vi "Periodic Tasks.vi"(8 "error in":errorcluster) -> ()   [LabVIEW 2013]
doc: "This VI runs in parallel to other tasks. It can contain as many user-defined periodic loops as you need. These can carry out PID or other sorts of timed response."
uses:
  <vilib>/Rock Robotics/SystemInterfaces/Utilities/FPGA_UtilitiesLED Source.ctl
  <vilib>/Rock Robotics/SystemInterfaces/Utilities/FPGA_UtilitiesLED State.ctl
  Robot Global Data.vi
panel:
  out "Value 2":bool
  out "Value":bool
  out "RDistance":dbl
  out "LDistance":dbl
  out "Distance":dbl
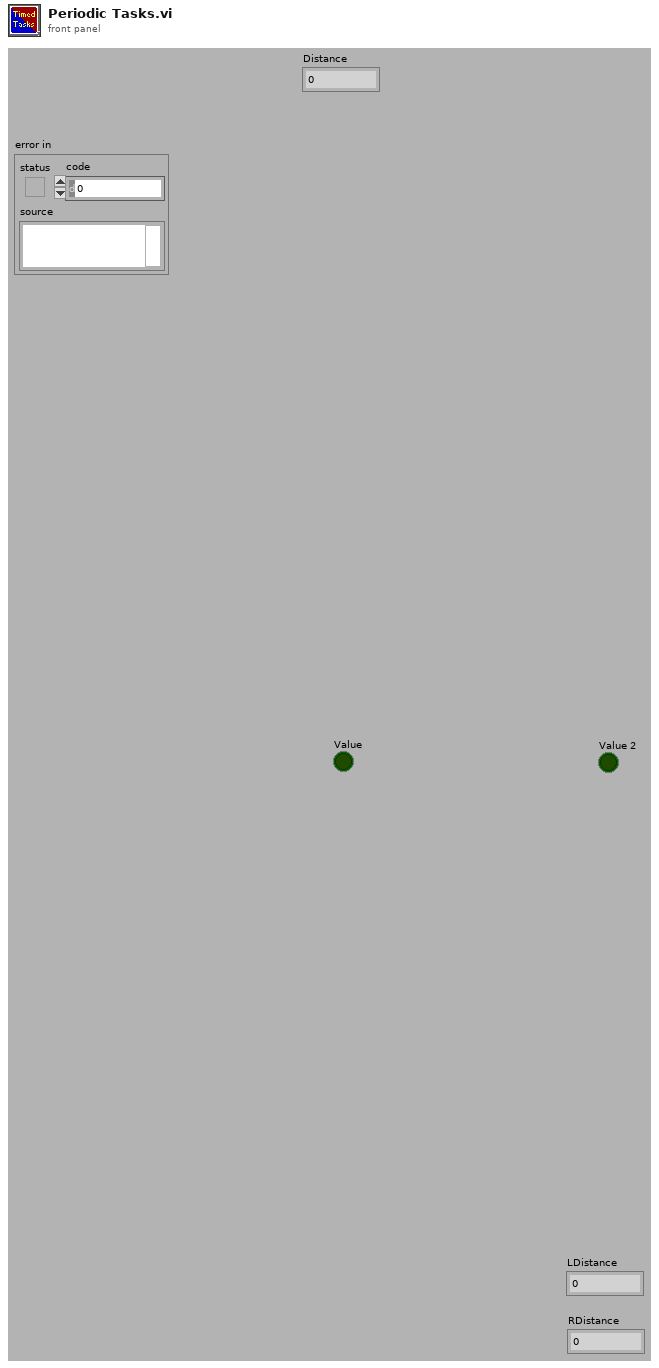
[diagram p1: front panel]
types:
  T1 = typedef "WPI_DigitalInputDevRef.ctl" = cluster{"DevStatus":errorcluster, "DIO Channel":T2, "Digital Module":T3}
  T2 = typedef "FPGA_DIOChannel.ctl" = enum8{"DIO 1", "DIO 2", "DIO 3", "DIO 4", "DIO 5", "DIO 6", "DIO 7", "DIO 8", "DIO 9", "DIO 10", "DIO 11", "DIO 12", "DIO 13", "DIO 14", "Invalid"}
  T3 = typedef "FPGA_TypedefDigitalModule.ctl" = enum16{"Digital Module 1", "Digital Module 2"}
  T4 = typedef "WPI_AnalogChannelDevRef.ctl" = cluster{"DevStatus":errorcluster, "Analog Module":T5, "Analog Channel":T6}
  T5 = typedef "FPGA_TypedefAnalogModule.ctl" = enum16{"Analog Module 1", "Analog Module 2"}
  T6 = typedef "FPGA_AIChannel.ctl" = enum8{"AI 1", "AI 2", "AI 3", "AI 4", "AI 5", "AI 6", "AI 7", "AI 8", "Invalid"}
  T7 = typedef "WPI_EncoderDevRef.ctl" = cluster{"DevStatus":errorcluster, "EncoderIndex":T8, "CounterIndex":T9, "DistancePerCount":dbl, "Decoding Type":T10}
  T8 = typedef "FPGA_EncoderIdx.ctl" = enum8{"Enc 0", "Enc 1", "Enc 2", "Enc 3", "Invalid"}
  T9 = typedef "FPGA_CounterCtrSystemIndex.ctl" = enum8{"Ctr 0", "Ctr 1", "Ctr 2", "Ctr 3", "Ctr 4", "Ctr 5", "Ctr 6", "Ctr 7", "Invalid"}
  T10 = typedef "WPI_EncoderType.ctl" = enum16{"1x", "2x", "4x"}
  T11 = cluster{"Winch Desired Location":dbl, "Winch Desired Location 2":dbl, "Winch Desired Location 3":dbl}
  T12 = typedef "FPGA_UtilitiesLED State.ctl" = enum16{"Off", "On", "Toggle"}
  T13 = typedef "FPGA_UtilitiesLED Source.ctl" = enum16{"User LED", "FPGA LED"}
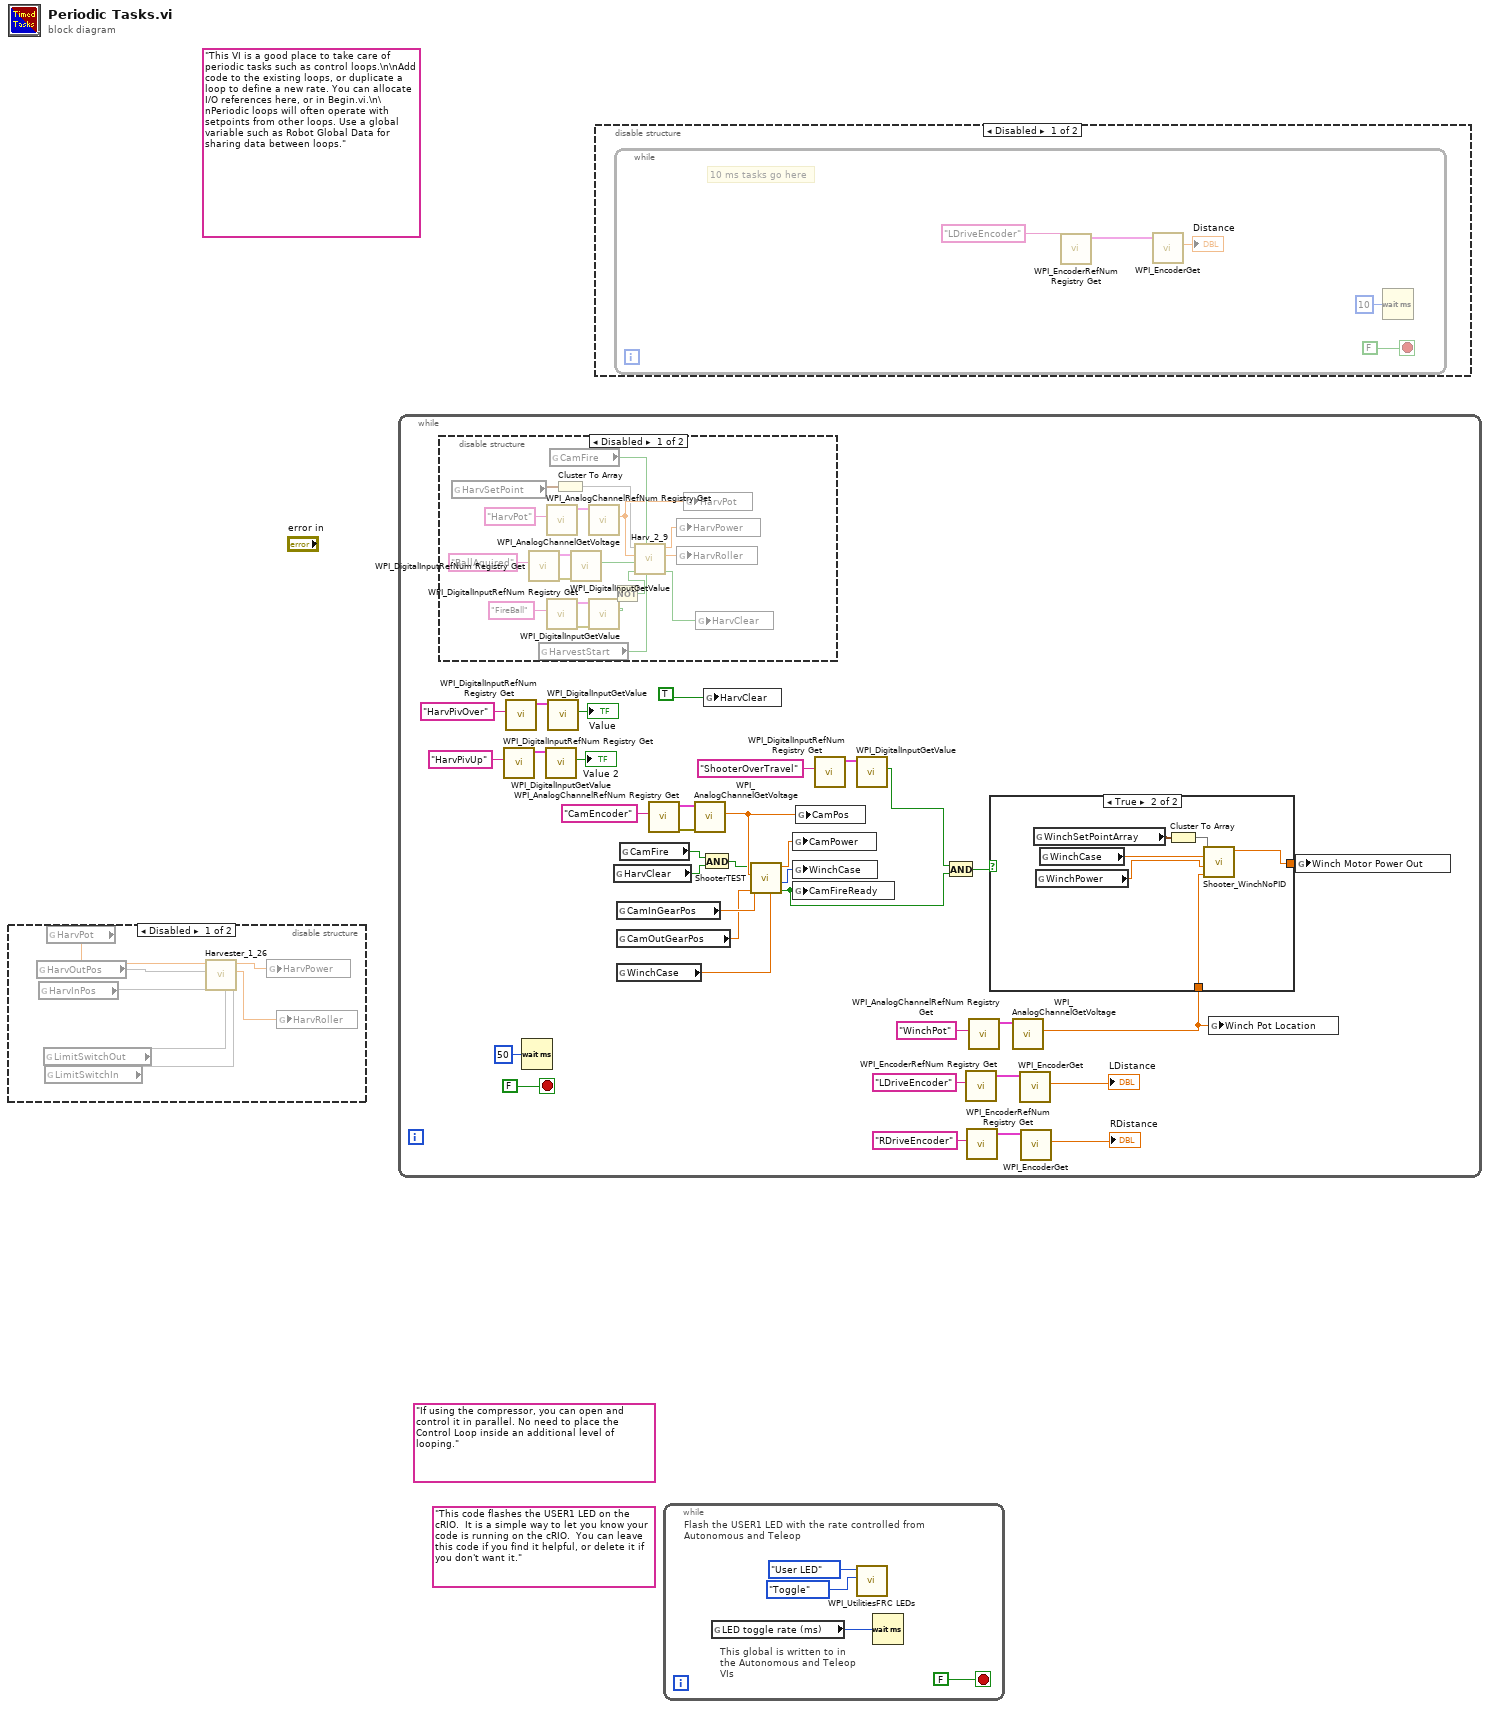
[diagram p0: block diagram]
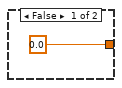
[diagram p5: hidden frame]
diagram:
  (unwired) "If using the compressor, you can open and control it in parallel. No need to place the Control Loop inside an additional level of looping."
  (unwired) "This code flashes the USER1 LED on the cRIO.  It is a simple way to let you know your code is running on the cRIO.  You can leave this code if you find it helpful, or delete it if you don't want it."
  (unwired) "This VI is a good place to take care of periodic tasks such as control loops.\n\nAdd code to the existing loops, or duplicate a loop to define a new rate. You can allocate I/O references here, or in Begin.vi.\n\nPeriodic loops will often operate with setpoints from other loops. Use a global variable such as Robot Global Data for sharing data between loops."
  n1 = disable-structure shown="Disabled" {
    frame Disabled {
      n2 = global read "Robot Global Data.vi" "HarvOutPos"() -> (w6)
      n3 = global read "Robot Global Data.vi" "HarvInPos"() -> (w5)
      n4 = global read "Robot Global Data.vi" "LimitSwitchOut"() -> (w4)
      n5 = global read "Robot Global Data.vi" "LimitSwitchIn"() -> (w3)
      n6 = global read "Robot Global Data.vi" "HarvPot"() -> (w7:dbl)
      n7 = call "Harvester_1_26.vi"("LimitSwitchIn"=w3, "LimitSwitchOut"=w4, "HarvInPos"=w5, "HarvOutPos"=w6, "HarvPot"=w7) -> ("HarvRoller"=w2:dbl, "HarvPower"=w1:dbl)  [unwired: 5 in]
      n8 = global write "Robot Global Data.vi" "HarvPower"(w1) -> ()
      n9 = global write "Robot Global Data.vi" "HarvRoller"(w2) -> ()
    }
    frame Enabled {
    }
  }
  n10 = while {
    stop <- FALSE stop-if-true
    n11 = disable-structure shown="Disabled" {
      frame Disabled {
        n12 = global read "Robot Global Data.vi" "HarvSetPoint"() -> (w45:cluster{"Out":dbl, "In":dbl, "Clear":dbl})
        n13 = call <vilib>:"WPI_DigitalInputRefNum Registry Get.vi"("refnum name"="BallAquired") -> ("error out"=w62:errorcluster, "DigitalInputDevRef"=w61:T1)  [unwired: 9 in]
        n14 = global read "Robot Global Data.vi" "HarvestStart"() -> (w51:bool)
        n15 = call <vilib>:"WPI_AnalogChannelRefNum Registry Get.vi"("refnum name"="HarvPot") -> ("AIDeviceRef"=w57:T4)  [unwired: 9 in, 1 out]
        n16 = call <vilib>:"WPI_DigitalInputRefNum Registry Get.vi"("refnum name"="FireBall") -> ("error out"=w53:errorcluster, "DigitalInputDevRef"=w54:T1)  [unwired: 9 in]
        n17 = global read "Robot Global Data.vi" "CamFire"() -> (w52:bool)
        n18 = Cluster To Array(cluster=w45) -> (array=w44:dbl[])
        n19 = call <vilib>:"WPI_DigitalInputGetValue.vi"("error in (no error)"=w62, "DigitalInputDevRef"=w61) -> ("Value"=w47:bool)  [unwired: 7 in, 2 out]
        n20 = call <vilib>:"WPI_AnalogChannelGetVoltage.vi"("AIDeviceRef"=w57) -> ("Voltage"=w50:dbl)  [unwired: 8 in, 2 out]
        n21 = call <vilib>:"WPI_DigitalInputGetValue.vi"("error in (no error)"=w53, "DigitalInputDevRef"=w54) -> ("Value"=w49:bool)  [unwired: 7 in, 2 out]
        n22 = Not(x=w49) -> (.not. x?=w46:bool)
        n23 = call "Harv_2_9.vi"("Harvest"=w51, "Fire"=w52, "FireBallSen"=w46, "BallAcquired"=w47, "HarvPot"=w50, "HarvSetpoints"=w44) -> ("HarvCleared"=w48:bool, "HarvRoller"=w58:dbl, "HarvPower"=w59:dbl)  [unwired: 3 in]
        n24 = global write "Robot Global Data.vi" "HarvPower"(w59) -> ()
        n25 = global write "Robot Global Data.vi" "HarvRoller"(w58) -> ()
        n26 = global write "Robot Global Data.vi" "HarvPot"(w50) -> ()
        n27 = global write "Robot Global Data.vi" "HarvClear"(w48) -> ()
      }
      frame Enabled {
      }
    }
    n28 = call <vilib>:"WPI_DigitalInputRefNum Registry Get.vi"("refnum name"="HarvPivUp") -> ("DigitalInputDevRef"=w14:T1)  [unwired: 9 in, 1 out]
    n29 = call <vilib>:"WPI_DigitalInputRefNum Registry Get.vi"("refnum name"="HarvPivOver") -> ("DigitalInputDevRef"=w32:T1)  [unwired: 9 in, 1 out]
    n30 = Wait (ms)(milliseconds to wait=u32 50) -> ()  [unwired: 1 out]
    n31 = call <vilib>:"WPI_DigitalInputGetValue.vi"("DigitalInputDevRef"=w14) -> ("Value"=→"Value 2":bool)  [unwired: 8 in, 2 out]
    n32 = call <vilib>:"WPI_DigitalInputGetValue.vi"("DigitalInputDevRef"=w32) -> ("Value"=→"Value":bool)  [unwired: 8 in, 2 out]
    n33 = global read "Robot Global Data.vi" "HarvClear"() -> (w21:bool)
    n34 = global read "Robot Global Data.vi" "CamInGearPos"() -> (w29:dbl)
    n35 = global read "Robot Global Data.vi" "CamOutGearPos"() -> (w28:dbl)
    n36 = global read "Robot Global Data.vi" "WinchCase"() -> (w22:dbl)
    n37 = global read "Robot Global Data.vi" "CamFire"() -> (w20:bool)
    n38 = call <vilib>:"WPI_AnalogChannelRefNum Registry Get.vi"("refnum name"="CamEncoder") -> ("error out"=w26:errorcluster, "AIDeviceRef"=w25:T4)  [unwired: 9 in]
    n39 = call <vilib>:"WPI_AnalogChannelGetVoltage.vi"("error in (no error)"=w26, "AIDeviceRef"=w25) -> ("Voltage"=w24:dbl)  [unwired: 7 in, 2 out]
    n40 = And(x=w20, y=w21) -> (x .and. y?=w19:bool)
    n41 = global write "Robot Global Data.vi" "HarvClear"(TRUE ("HarvClear")) -> ()
    n42 = call "ShooterTEST.vi"("WinchCaseIn"=w22, "OutGearPos"=w28, "InGearPos"=w29, "Pot"=w24, "Fire"=w19) -> ("There?"=w10:bool, "WinchCase"=w23:i32, "Power"=w18:dbl)  [unwired: 4 in]
    n43 = global write "Robot Global Data.vi" "CamPower"(w18) -> ()
    n44 = global write "Robot Global Data.vi" "WinchCase"(w23) -> ()
    n45 = global write "Robot Global Data.vi" "CamFireReady"(w10) -> ()
    n46 = global write "Robot Global Data.vi" "CamPos"(w24) -> ()
    n47 = call <vilib>:"WPI_DigitalInputRefNum Registry Get.vi"("refnum name"="ShooterOverTravel") -> ("DigitalInputDevRef"=w13:T1)  [unwired: 9 in, 1 out]
    n48 = call <vilib>:"WPI_DigitalInputGetValue.vi"("DigitalInputDevRef"=w13) -> ("Value"=w9:bool)  [unwired: 8 in, 2 out]
    n49 = And(x=w9, y=w10) -> (x .and. y?=w11:bool)
    n50 = call <vilib>:"WPI_EncoderRefNum Registry Get.vi"("refnum name"="LDriveEncoder") -> ("EncoderDevRef"=w37:T7)  [unwired: 9 in, 1 out]
    n51 = call <vilib>:"WPI_EncoderRefNum Registry Get.vi"("refnum name"="RDriveEncoder") -> ("EncoderDevRef"=w34:T7)  [unwired: 9 in, 1 out]
    n52 = call <vilib>:"WPI_AnalogChannelRefNum Registry Get.vi"("refnum name"="WinchPot") -> ("AIDeviceRef"=w40:T4)  [unwired: 9 in, 1 out]
    n53 = call <vilib>:"WPI_AnalogChannelGetVoltage.vi"("AIDeviceRef"=w40) -> ("Voltage"=w39:dbl)  [unwired: 8 in, 2 out]
    n54 = case shown="True" w11 {
      tunnel: [0.0 ("Winch Motor Power Out") w65] -> w30
      tunnel: w39 -> [_ w66]
      frame False {
      }
      frame True {
        n55 = global read "Robot Global Data.vi" "WinchSetPointArray"() -> (w68:T11)
        n56 = global read "Robot Global Data.vi" "WinchPower"() -> (w64:dbl)
        n57 = global read "Robot Global Data.vi" "WinchCase"() -> (w69:dbl)
        n58 = Cluster To Array(cluster=w68) -> (array=w67:dbl[])
        n59 = call "Shooter_WinchNoPID.vi"("Winch Pot Location"=w66, "WinchPower"=w64, "selectedCase"=w69, "SetPointArray"=w67) -> ("Winch Motor Power Out"=w65:dbl)  [unwired: 7 in]
      }
    }
    n60 = call <vilib>:"WPI_EncoderGet.vi"("EncoderDevRef"=w37) -> ("Distance"=→"LDistance":dbl)  [unwired: 5 in, 5 out]
    n61 = call <vilib>:"WPI_EncoderGet.vi"("EncoderDevRef"=w34) -> ("Distance"=→"RDistance":dbl)  [unwired: 5 in, 5 out]
    n62 = global write "Robot Global Data.vi" "Winch Pot Location"(w39) -> ()
    n63 = global write "Robot Global Data.vi" "Winch Motor Power Out"(w30) -> ()
  }
  n64 = disable-structure shown="Disabled" {
    frame Disabled {
      n65 = while {
        stop <- FALSE stop-if-true
        # "10 ms tasks go here"
        n66 = call <vilib>:"WPI_EncoderRefNum Registry Get.vi"("refnum name"="LDriveEncoder") -> ("EncoderDevRef"=w70:T7)  [unwired: 9 in, 1 out]
        n67 = call <vilib>:"WPI_EncoderGet.vi"("EncoderDevRef"=w70) -> ("Distance"=→"Distance":dbl)  [unwired: 5 in, 5 out]
        n68 = Wait (ms)(milliseconds to wait=u32 10) -> ()  [unwired: 1 out]
      }
    }
    frame Enabled {
    }
  }
  n69 = while {
    stop <- FALSE stop-if-true
    # "This global is written to in the Autonomous and Teleop VIs"
    # "Flash the USER1 LED with the rate controlled from Autonomous and Teleop"
    n70 = global read "Robot Global Data.vi" "LED toggle rate (ms)"() -> (w75:u32)
    n71 = call <vilib>:"WPI_UtilitiesFRC LEDs.vi"("State"=FPGA_UtilitiesLED_State."Toggle", "LED Type"=FPGA_UtilitiesLED_Source."User LED") -> ()  [unwired: 1 in, 9 out]
    n72 = Wait (ms)(milliseconds to wait=w75) -> ()  [unwired: 1 out]
  }
